vi "Package Source.vi"(8 "error in (no error)":errorcluster, 11 "PackageInfo in":refnum<class "PackageInfo.lvclass">) -> (0 "error out":errorcluster, 2 "Package Source":string)   [LabVIEW 2020, in "GPack.lvlib" / "PackageInfo.lvclass"]
uses:
  PackageInfo.lvclass
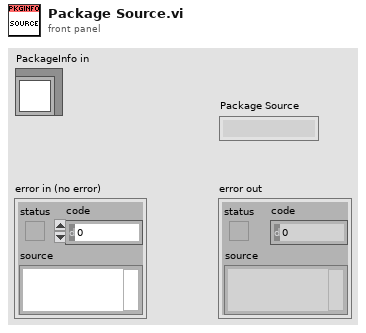
[diagram p1: front panel]
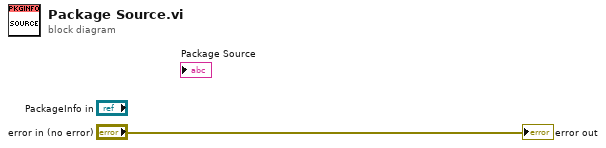
[diagram p0: block diagram]
diagram:
  "error out" <- "error in (no error)"
